vi "Find_Average.vi"() -> ()   [LabVIEW 2010]
uses:
  <vilib>/express/express arith-compare/Formula/XNode/ExpressFormulaBlockNode.xnode
panel:
  in  "stop":bool
  out "Average":dbl
  in  "Number 3":dbl
  in  "Number 2":dbl
  in  "Number 1":dbl
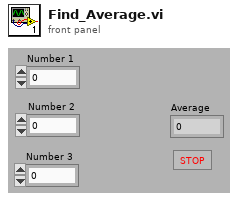
[diagram p1: front panel]
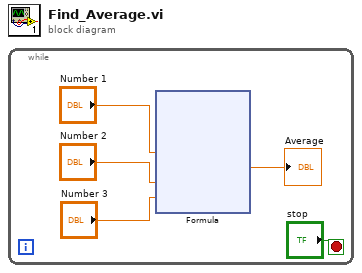
[diagram p0: block diagram]
diagram:
  n1 = while {
    stop <- "stop" stop-if-true
    n2 = xnode "Formula"("X1"="Number 1", "X2"="Number 2", "X3"="Number 3") -> ("Result"=→"Average":dbl)  [unwired: 1 in, 1 out]
  }
